vi "util.file.record.load.vi"(8 "error in":errorcluster, 11 "filename.*":string) -> (0 "error out":errorcluster, 2 "Multiple Plots (X Array and Y Array)":cluster{"all rows":dbl[], "all rows":dbl[]}(graph), 3 "Multiple Plots (X Array and Y Array) 2":cluster{"X":dbl[], "Y":dbl[]})   [LabVIEW 2024]
doc: "Illustrates the various data types that the XY Graph accepts. Use the XY Graph to display data that is not uniformly distributed along the X-axis. This is particularly useful when displaying data that was sampled at a variable rate. The XY Graph is also useful for displaying data that is formatted as (X,Y) pairs."
uses:
  controls/typePathSelector.ctl
  <vilib>/Utility/error.llb/Clear Errors.vi
  <vilib>/Utility/libraryn.llb/Create Directory Recursive.vi
  <vilib>/Utility/file.llb/Read Delimited Spreadsheet (DBL).vi
panel:
  out "new file path (Not A Path if cancelled)":path
  # "example: \nfolder1\\folder2\\filename.log"
  # "folder1\\folder2\\..\\folderN\\file.log"
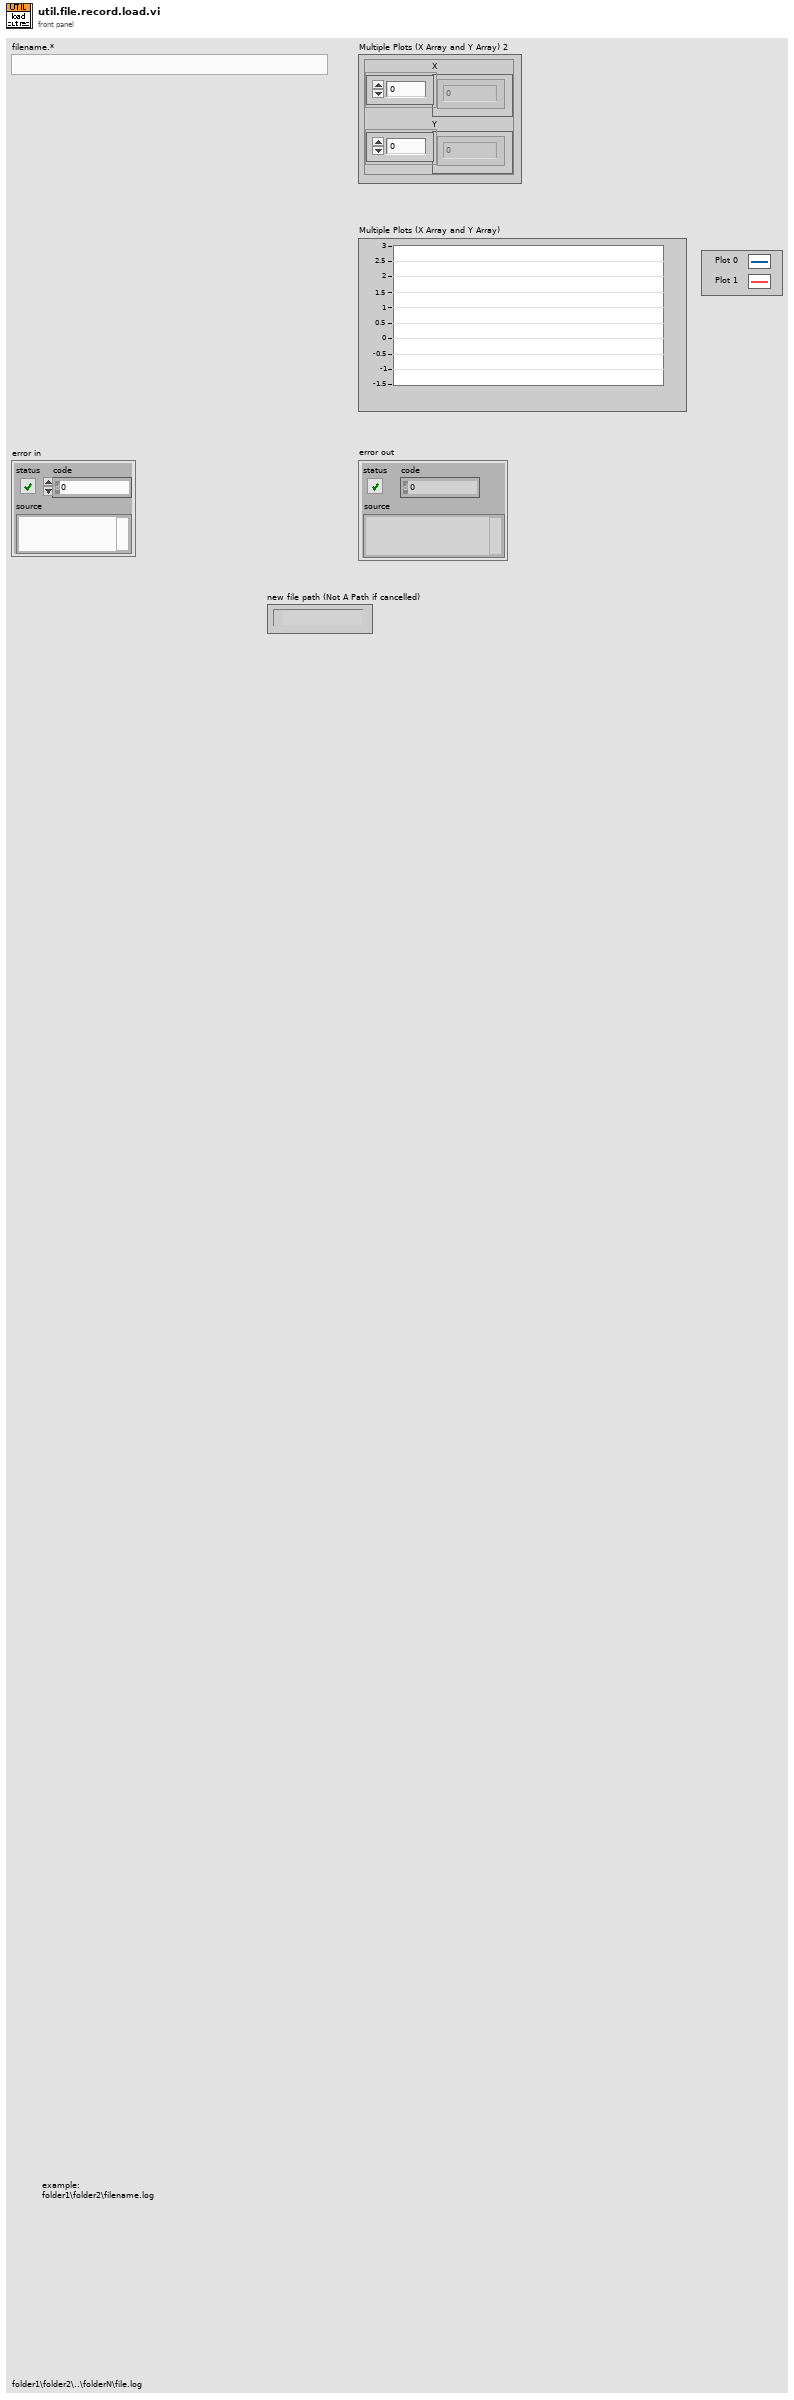
[diagram p1: front panel]
types:
  T1 = typedef "typePathSelector.ctl" = enum16{"DIR_PROCS", "DIR_CONFIG", "DIR_TEMPLATE", "DIR_IO_FILE", "DIR_RECORD", "DIR_LOG", "DIR_RUNTIME", "DIR_PRESET", "DIR_INI"}
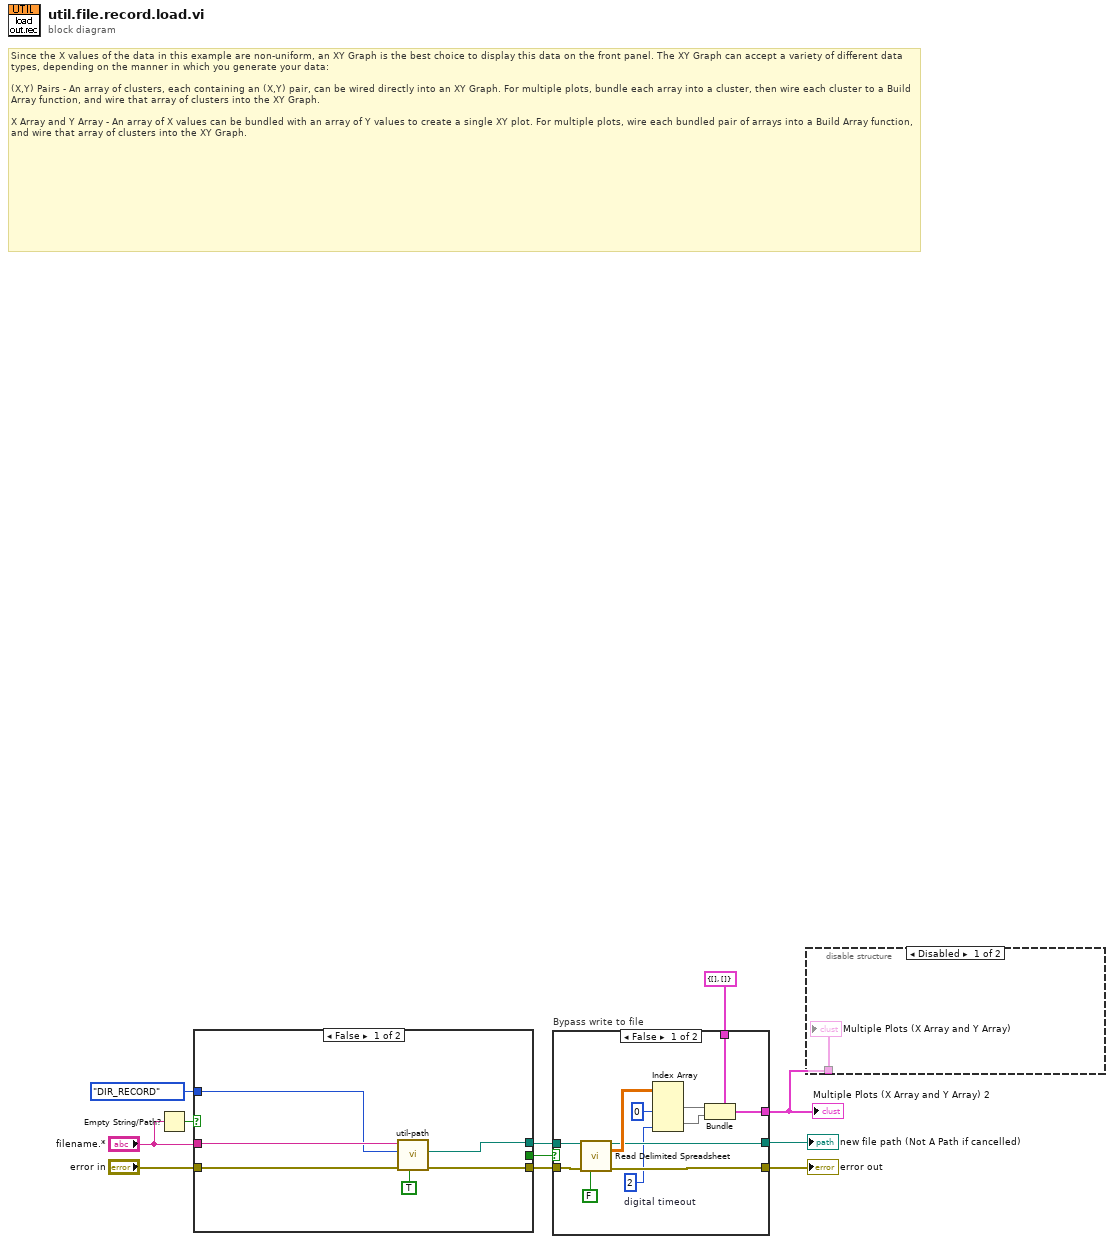
[diagram p0: block diagram]
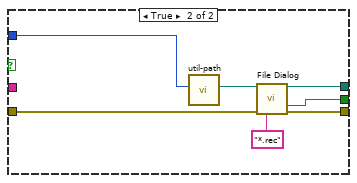
[diagram p4: hidden frame]
diagram:
  # "Since the X values of the data in this example are non-uniform, an XY Graph is the best choice to display this data on the front panel. The XY Graph can accept a variety of different data types, depending on the manner in which you generate your data:\n\n(X,Y) Pairs - An array of clusters, each containing an (X,Y) pair, can be wired directly into an XY Graph. For multiple plots, bundle each array into a cluster, then wire each cluster to a Build Array function, and wire that array of clusters into the XY Graph.\n\nX Array and Y Array - An array of X values can be bundled with an array of Y values to create a single XY plot. For multiple plots, wire each bundled pair of arrays into a Build Array function, and wire that array of clusters into the XY Graph."
  n1 = Empty String/Path?(string/path="filename.*") -> (empty?=w11:bool)
  n2 = case shown="False" w11 {
    tunnel: [w13 w24] -> w8
    tunnel: "error in" -> [w14 w23]
    tunnel: [w15 w22] -> w9
    tunnel: "filename.*" -> [w17 _]
    tunnel: [_ w19] -> w7
    tunnel: typePathSelector."DIR_RECORD" ("Enum") -> [w12 w18]
    frame False {
      n3 = call "util-path.vi"("Create Folders?(F)"=TRUE, "error in"=w14, "Selected Folder (PROCS)"=w12, "append path (ie. folder\\filename.*)"=w17) -> ("error out"=w13:errorcluster, "SelectedPath"=w15:path)  [unwired: 3 in, 3 out]
    }
    frame True {
      n4 = call "util-path.vi"("Selected Folder (PROCS)"=w18) -> ("SelectedPath"=w21:path)  [unwired: 6 in, 4 out]
      n5 = call "File Dialog"("start path"=w21, "error in"=w23, "pattern (all files)"="*.rec") -> ("selected path"=w22:path, "cancelled"=w19:bool, "error out"=w24:errorcluster)  [unwired: 9 in, 1 out]
    }
  }
  n6 = case "Bypass write to file" shown="False" w7 {
    tunnel: w9 -> [w32 _]
    tunnel: w8 -> [w31 w38]
    tunnel: [w30 w37] -> w1
    tunnel: [w29 w38] -> w6
    tunnel: [w28 _] -> w3
    tunnel: cluster{"X":dbl[], "Y":dbl[]} {"X"=[], "Y"=[]} ("Multiple Plots (X Array and Y Array)") -> [w25 w37]
    frame False {
      w26 = 2  # digital timeout
      n7 = call-poly <vilib>:"Read Delimited Spreadsheet.vi"("file path (dialog if empty)"=w32, "error in (no error)"=w31, "transpose? (F)"=FALSE) -> ("new file path (Not A Path if cancelled)"=w28:path, "all rows"=w33:dbl[][], "error out"=w29:errorcluster)  [unwired: 7 in, 3 out]
      n8 = Index Array(array=w33, index (col) #1=0 ("disabled index (col)"), index (col) #2=w26) -> (element #1=w35:dbl[], element #2=w36:dbl[])  [unwired: 2 in]
      n9 = Bundle(cluster=w25, "X"=w35, "Y"=w36) -> (w30:cluster{"X":dbl[], "Y":dbl[]})
    }
    frame True {
    }
  }
  "error out" <- w6
  "new file path (Not A Path if cancelled)" <- w3
  "Multiple Plots (X Array and Y Array) 2" <- w1
  n10 = disable-structure shown="Disabled" {
    disable-tunnel: w1 -> [w39 _]
    frame Disabled {
      "Multiple Plots (X Array and Y Array)" <- w39
    }
    frame Enabled {
    }
  }
